vi "Package stage data to cluster.vi"(7 "axis":u32=2, 8 "error in (no error)":errorcluster, 9 "Increasement":dbl format="%#_13g", 10 "relative?":bool=TRUE, 11 "direction":bool=TRUE) -> (0 "error out":errorcluster, 3 "Stage Ctrl":T1)   [LabVIEW 2020]
doc: "Generates sample waveforms according to the signal type in the HW Config input."
uses:
  Stage Ctrl.ctl
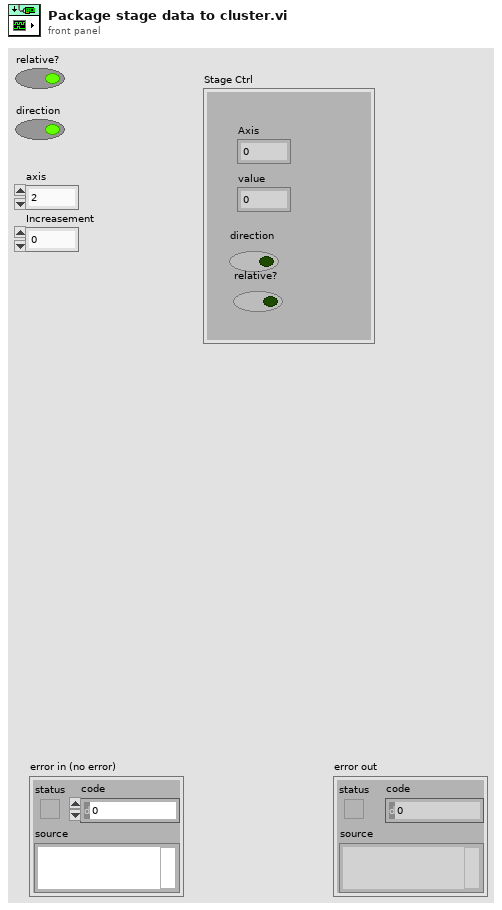
[diagram p1: front panel]
types:
  T1 = typedef "Stage Ctrl.ctl" = cluster{"Axis":dbl, "value":dbl, "direction":bool, "relative?":bool}
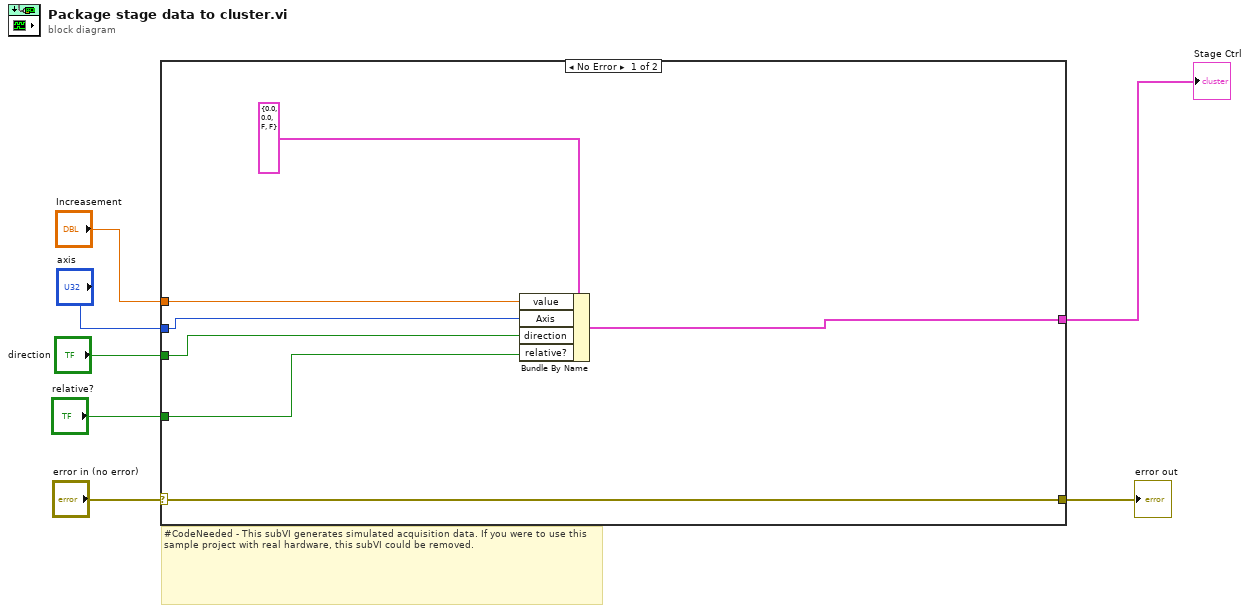
[diagram p0: block diagram]
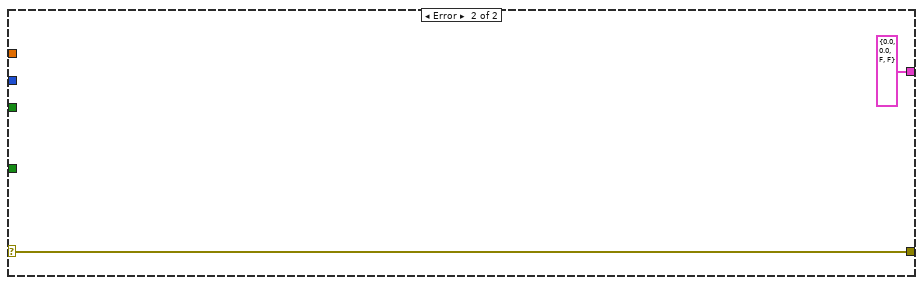
[diagram p2: hidden frame]
diagram:
  # "#CodeNeeded - This subVI generates simulated acquisition data. If you were to use this sample project with real hardware, this subVI could be removed."
  n1 = case shown="No Error" "error in (no error)" {
    selector: "error in (no error)" -> [w14 w16]
    tunnel: [w14 w16] -> w6
    tunnel: "axis" -> [w11 _]
    tunnel: "Increasement" -> [w12 _]
    tunnel: "direction" -> [w10 _]
    tunnel: [w9 T1 {"Axis"=0.0, "value"=0.0, "direction"=FALSE, "relative?"=FALSE} ("Stage Ctrl")] -> w2
    tunnel: "relative?" -> [w8 _]
    frame No Error {
      n2 = Bundle By Name(cluster=T1 {"Axis"=0.0, "value"=0.0, "direction"=FALSE, "relative?"=FALSE} ("Stage Ctrl"), "value"=w12, "Axis"=w11, "direction"=w10, "relative?"=w8) -> (w9:T1)
    }
    frame Error {
    }
  }
  "error out" <- w6
  "Stage Ctrl" <- w2
